vi "StringToSSM.vi"(6 "Last Command (Stop)":string="Stop", 7 "Bus Reference":refnum<class "Bus.lvclass">, 8 "Error Out":errorcluster, 9 "Test Index (0)":i32, 10 "ModuleList":string[](array[string]), 11 "SSM Case":string="RunTest") -> (0 "Error Out 2":errorcluster, 2 "SSM Array":string[](array[string]), 3 "TestClass":refnum<class "Test.lvclass">)   [LabVIEW 2018]
doc: "This VI sends a message to loads the new plugin into the module."
uses:
  NistPluggableModules/BusClass/Bus.lvclass
  NistPluggableModules/TestClass/Test.lvclass
  NistPluggableModules/BusClass/Bus.lvclass/Bus.ctl
  NistPluggableModules/BusClass/Accessors/Read Test.vi
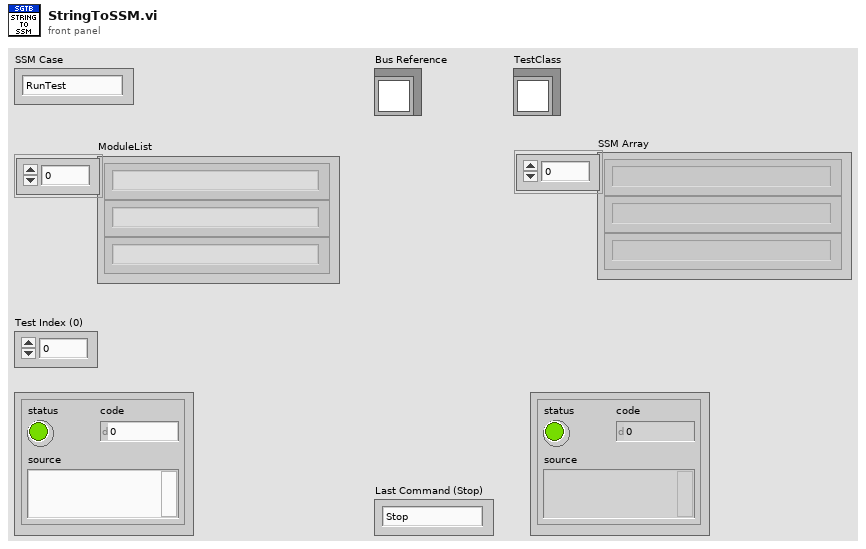
[diagram p1: front panel]
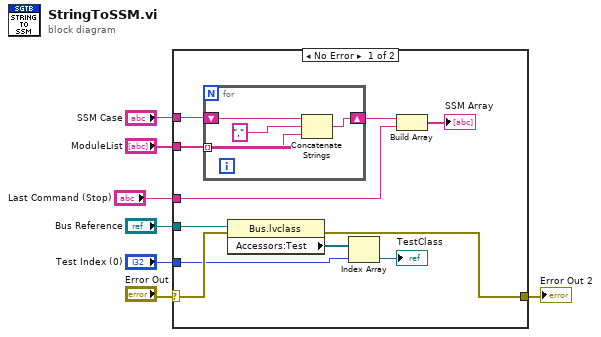
[diagram p0: block diagram]
diagram:
  n1 = case shown="No Error" "Error Out" {
    selector: "Error Out" -> [w13 w23]
    tunnel: "ModuleList" -> [w17 _]
    tunnel: "SSM Case" -> [w16 _]
    tunnel: [w10 w23] -> w4
    tunnel: "Test Index (0)" -> [w12 _]
    tunnel: "Bus Reference" -> [w11 _]
    tunnel: "Last Command (Stop)" -> [w8 _]
    frame No Error {
      n2 = for {
        tunnel: w17 -> [w19] mode=indexing
        shift-right: [w21] -> w18
        shift-left: w16 -> [w22]
        n3 = Concatenate Strings(w22, "," ("string"), w19) -> (w21:string)
      }
      n4 = property class="Bus.lvclass"(reference=w11, error in=w13) -> (error out=w10:errorcluster, "Accessors:Test"=w14:refnum<class "Test.lvclass">[])  [unwired: 1 out]
      n5 = Index Array(array=w14, index=w12) -> (element=→"TestClass":refnum<class "Test.lvclass">)
      n6 = Build Array(w18, w8) -> (→"SSM Array":string[])
    }
    frame Error {
    }
  }
  "Error Out 2" <- w4
